vi "sub_rolling average.vi"(5 "Raw Data":u16[][](array[numeric]), 8 "错误输入（无错误）":errorcluster, 9 "队列输入":refnum<queue>, 10 "移位in":dbl[][](array[numeric]), 11 "Image Create":T1) -> (0 "错误输出":errorcluster, 1 "队列输出":refnum<queue>, 2 "移位out":dbl[][](array[numeric]), 3 "Image Display":T1, 4 "队列中元素数量":i32)   [LabVIEW 2015]
uses:
  <vilib>/vision/Image Controls.llb/IMAQ Image.ctl
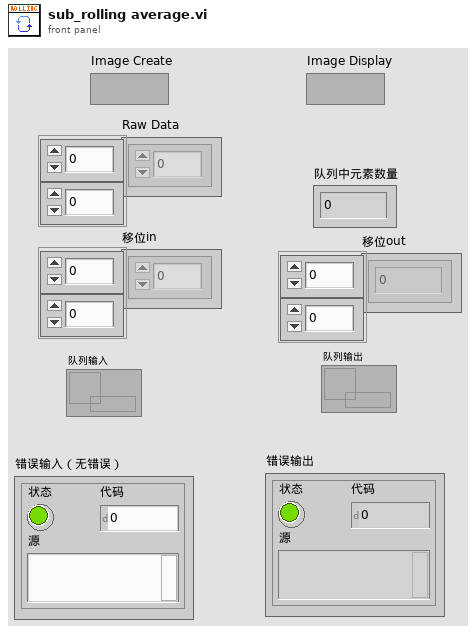
[diagram p1: front panel]
types:
  T1 = typedef "IMAQ Image.ctl" = refnum<image>
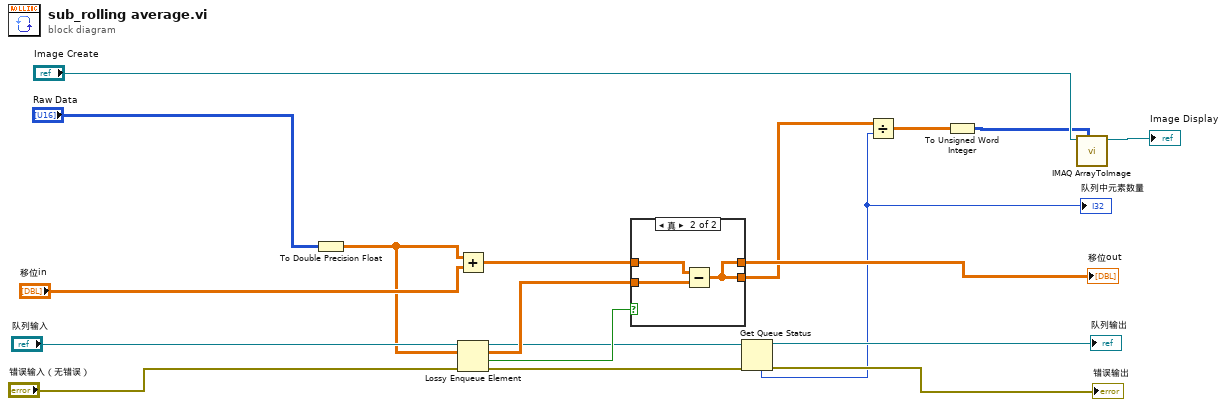
[diagram p0: block diagram]
diagram:
  n1 = To Double Precision Float(number="Raw Data") -> (double precision float=w5:dbl[][])
  n2 = Add(x=w5, y="移位in") -> (x+y=w9:dbl[][])
  n3 = Lossy Enqueue Element(queue="队列输入", element=w5, error in (no error)="错误输入（无错误）") -> (queue out=w6:refnum<queue>, overflow element=w8:dbl[][], overflow?=w7:bool, error out=w2:errorcluster)
  n4 = case shown="真" w7 {
    tunnel: w8 -> [_ w23]
    tunnel: w9 -> [w20 w22]
    tunnel: [w20 w21] -> w3
    tunnel: [w20 w21] -> w18
    frame False {
    }
    frame True {
      n5 = Subtract(x=w22, y=w23) -> (x-y=w21:dbl[][])
    }
  }
  "移位out" <- w18
  n6 = Get Queue Status(queue=w6, error in (no error)=w2) -> (queue out=→"队列输出":refnum<queue>, error out=→"错误输出":errorcluster, # elements in queue=w11:i32)  [unwired: 1 in, 5 out]
  "队列中元素数量" <- w11
  n7 = Divide(x=w3, y=w11) -> (x/y=w4:dbl[][])
  n8 = To Unsigned Word Integer(number=w4) -> (unsigned 16bit integer=w1:u16[][])
  n9 = call "IMAQ ArrayToImage"("Image Pixels (U16)"=w1, "Image"="Image Create") -> ("Image Out"=→"Image Display":T1)  [unwired: 8 in, 1 out]
